vi "Write Data Size.vi"(8 "error in":errorcluster, 10 "data size":i32=19, 11 "ARINC 429 in":refnum<class "ARINC 429.lvclass">) -> (0 "error out":errorcluster, 3 "ARINC 429 out":refnum<class "ARINC 429.lvclass">)   [LabVIEW 2020, in "ARINC 429.lvclass"]
uses:
  ARINC 429.lvclass
  ARINC 429.lvclass/ARINC 429.ctl
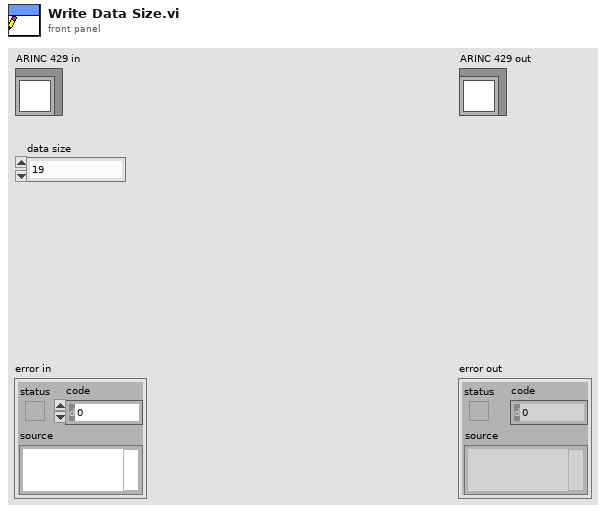
[diagram p1: front panel]
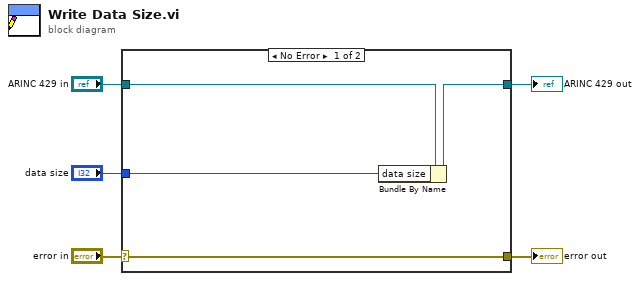
[diagram p0: block diagram]
diagram:
  n1 = case shown="No Error" "error in" {
    selector: "error in" -> [w9 w10]
    tunnel: [w9 w10] -> w4
    tunnel: [w7 w11] -> w2
    tunnel: "ARINC 429 in" -> [w8 w11]
    tunnel: "data size" -> [w6 _]
    frame No Error {
      n2 = Bundle By Name(cluster=w8, "data size"=w6) -> (w7:refnum<class "ARINC 429.lvclass">)
    }
    frame Error {
    }
  }
  "error out" <- w4
  "ARINC 429 out" <- w2
